vi "Add Separator.vi"(8 "error in (no error)":errorcluster, 11 "TreeControl in":refnum<vi>) -> (0 "error out":errorcluster, 3 "TreeControl out":refnum<vi>)   [LabVIEW 2021, in "Seq Edit Quick Drop.lvlib"]
uses:
  Seq Edit Quick Drop.lvlib
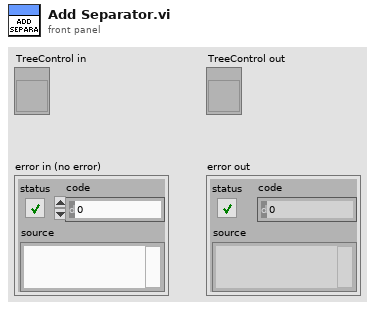
[diagram p1: front panel]
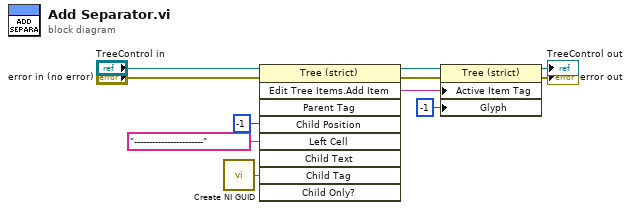
[diagram p0: block diagram]
diagram:
  n1 = call <vilib>:"Create NI GUID.vi"() -> ("NI GUID"=w10:string)
  n2 = invoke on="Invoke Node" class="Tree (strict)" method="Edit Tree Items.Add Item"(reference="TreeControl in", error in="error in (no error)", "Child Position"=-1, "Left Cell"="-----------------------" ("Left Cell String"), "Child Tag"=w10) -> (reference out=w6:refnum<vi>, error out=w4:errorcluster, "Edit Tree Items:Add Item"=w11:string)  [unwired: 4 in, 6 out]
  n3 = property class="Tree (strict)"(reference=w6, error in=w4, "Active Item Tag"=w11, "Glyph"=-1 ("Active Item:Symbol Index")) -> (reference out=→"TreeControl out":refnum<vi>, error out=→"error out":errorcluster)
